vi "Init.vi"(8 "error in (no error)":errorcluster, 11 "Configuration Window in":refnum<class "Configuration Window.lvclass">) -> (0 "error out":errorcluster, 3 "Configuration Window out":refnum<class "Configuration Window.lvclass">)   [LabVIEW 2018, in "Configuration Window.lvlib" / "Configuration Window.lvclass"]
uses:
  Configuration Window.lvclass
  Configuration Window.lvclass/Configuration Window.ctl
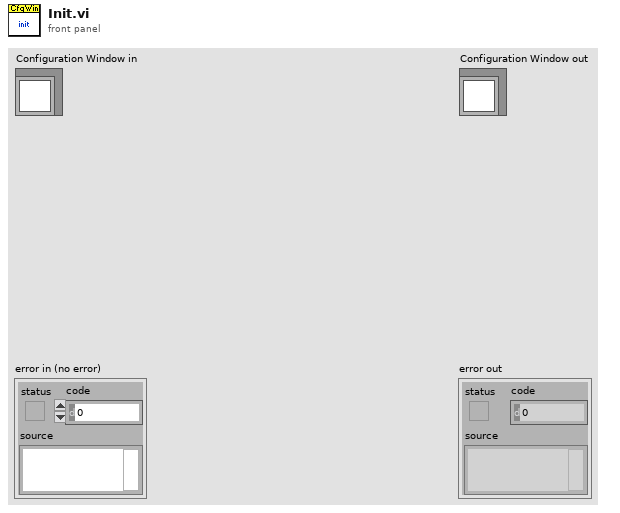
[diagram p1: front panel]
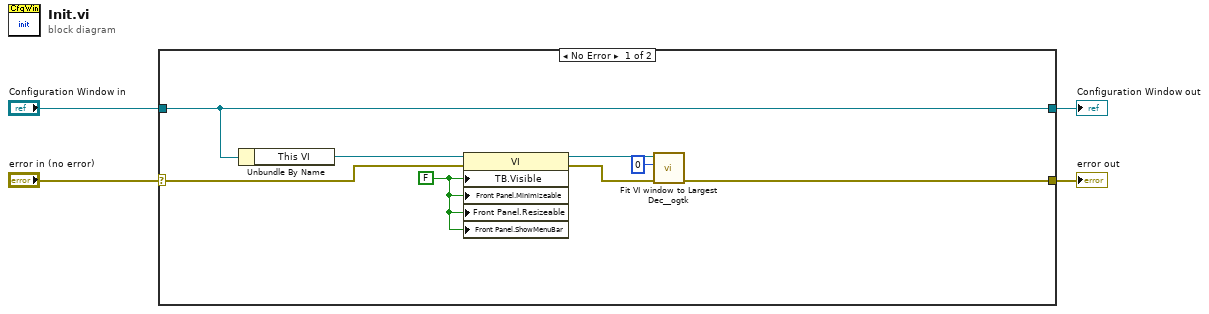
[diagram p0: block diagram]
diagram:
  n1 = case shown="No Error" "error in (no error)" {
    selector: "error in (no error)" -> [w9 w14]
    tunnel: [w6 w14] -> w3
    tunnel: [w12 w13] -> w1
    tunnel: "Configuration Window in" -> [w12 w13]
    frame No Error {
      w10 = FALSE ("Tool Bar:Visible")
      n2 = Unbundle By Name(w12) -> ("This VI"=w11:refnum<vi>)
      n3 = property class="VI"(reference=w11, error in=w9, "TB.Visible"=w10, "Front Panel.Minimizeable"=w10, "Front Panel.Resizeable"=w10, "Front Panel.ShowMenuBar"=w10) -> (reference out=w8:refnum<vi>, error out=w7:errorcluster)
      n4 = call <userlib>:"Fit VI window to Largest Dec__ogtk.vi"("error in (no error)"=w7, "border spacing (2 px)"=0, "VI Ref (calling VI)"=w8) -> ("error out"=w6:errorcluster)  [unwired: 3 in, 1 out]
    }
    frame Error {
    }
  }
  "error out" <- w3
  "Configuration Window out" <- w1
